vi "Set_Measurement_Conditions.vi"(3 "Simulate/Run":T3, 4 "Currently on Point":i32=11, 5 "Traverse line":T5 {"Row Duration (mins)" format="%#.1f"; "Row No" min=0; "Trace Gas Concentration (%)" min=0.0 format="%#.2f"; "Emission Rate (l/min)" format="%#.2f"; "Tunnel Speed" format="%#.2f"; "Start X" format="%#.2f"; "Start Y" format="%#.2f"; "Start Z" format="%#.2f"; "End X" format="%#.2f"; "End Y" format="%#.2f"; "End Z" format="%#.2f"; "Averaging time (min)" min=0.0 format="%#.2f"}) -> (0 "Status Cluster":T1)   [LabVIEW 2010]
uses:
  Traverse_cluster.ctl
  Spacing.ctl
  Controls/Multi_run_mode.ctl
  Execute_case.ctl
  Controls/User_Specific_mode.ctl
  Status_Cluster.ctl
  Multi_Run_Status.ctl
  ADAM Client/Sub VIs/ADAM Controls/Client_Source_Status.ctl
  Globals/Preference_global.vi
  Globals/Extra_Commands_Global.vi
panel:
  out "Heaters On?":bool
  out "Time Source Started":dbl
  out "Execute Case":T4=enum."Set All Conditions"
  # "X           Y            Z"
  # "Start"
  # "End"
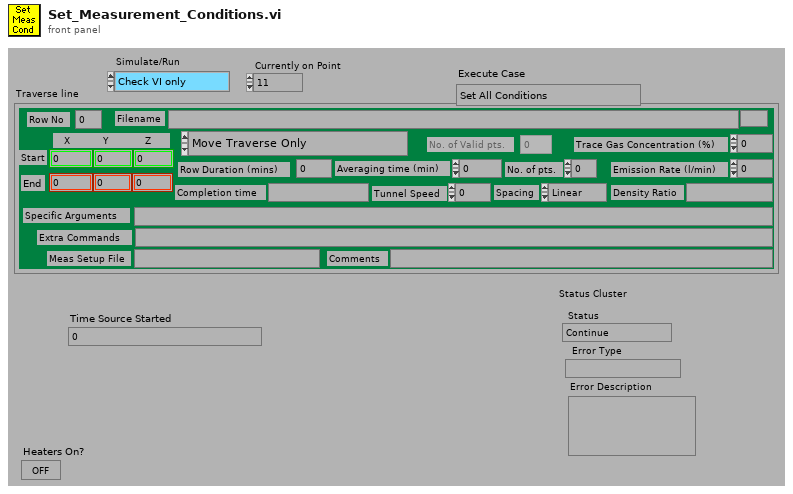
[diagram p1: front panel]
types:
  T1 = typedef "Status_Cluster.ctl" = cluster{"Status":T2, "Error Type":string, "Error Description":string}
  T2 = typedef "Multi_Run_Status.ctl" = enum16{"Continue", "Jump to Next Point", "Jump to Next Row", "Jump To Fall Back", "Terminate Run"}
  T3 = typedef "User_Specific_mode.ctl" = enum16{"Check VI only", "Run VI"}
  T4 = typedef "Execute_case.ctl" = enum16{"Start", "EnFlo Tunnel Check", "Set All Conditions", "Establish Exp Conditions", "The End"}
  T5 = typedef "Traverse_cluster.ctl" = cluster{"Start X":dbl, "Start Y":dbl, "Start Z":dbl, "End X":dbl, "End Y":dbl, "End Z":dbl, "No. of pts.":i32, "Spacing":T6, "Filename":path, "Tunnel Speed":dbl, "Averaging time (min)":dbl, "Extra Commands":string, "Specific Arguments":string, "Emission Rate (l/min)":dbl, "Trace Gas Concentration (%)":dbl, "Density Ratio":string, "Comments":string, "Row No":i32, "Row Type Selector":T7, "Completion time":string, "Row Duration (mins)":dbl, "No. of Valid pts.":i32, "Meas Setup File":string}
  T6 = typedef "Spacing.ctl" = enum16{"Linear", "Log", "Gauss", "Specified", "N/A"}
  T7 = typedef "Multi_run_mode.ctl" = enum16{"Move Traverse Only", "Set Tunnel Speed Only", "Set Source Only", "Set Measurement Conditions", "Single Measurement", "Vertical Profile", "Lateral Profile", "Longitudinal Profile", "Explore Volume", "Multi-Axis Profile", "Auto Calibrate", "Meas Fast FID Bkgnd", "Check Beam Power", "Scanning Valve Measurement", "Run VI Named:", "Set ADAM Ch", "Wait (minutes)", "Send Message", "Synchronize With:", "Fall Back to this Row", "Turn Off Row Repeating", "Blank Row"}
  T8 = typedef "Client_Source_Status.ctl" = enum16{"Not Using", "Using", "Must Have"}
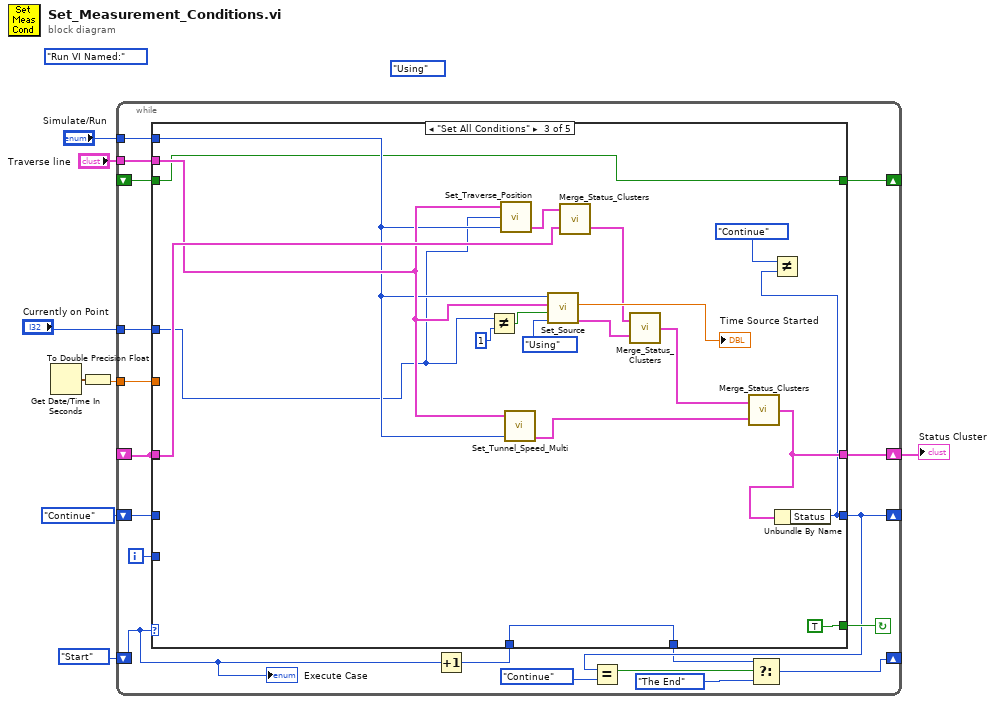
[diagram p0: block diagram]
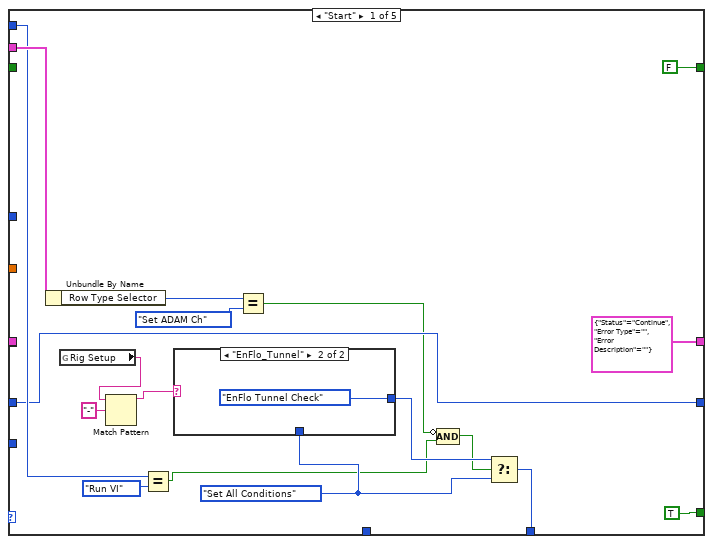
[diagram p2: hidden frame]
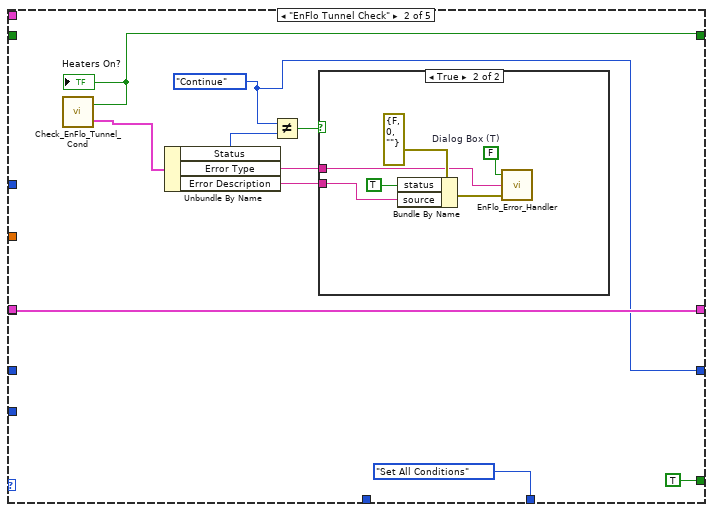
[diagram p4: hidden frame]
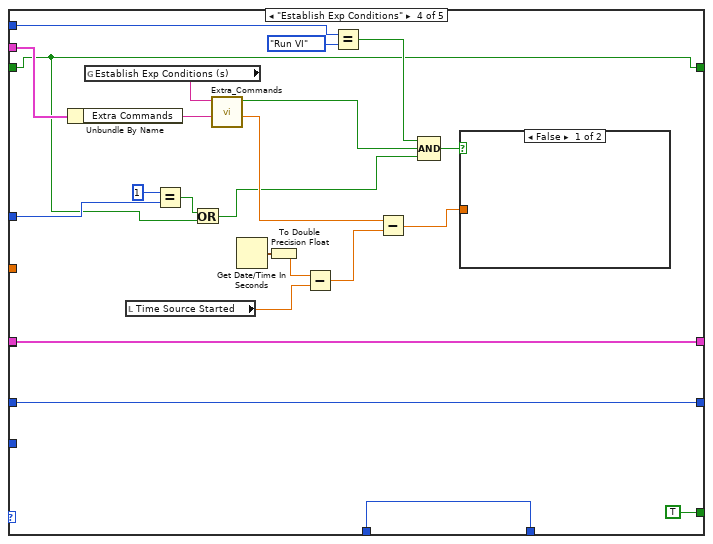
[diagram p6: hidden frame]
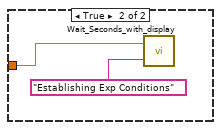
[diagram p7: hidden frame]
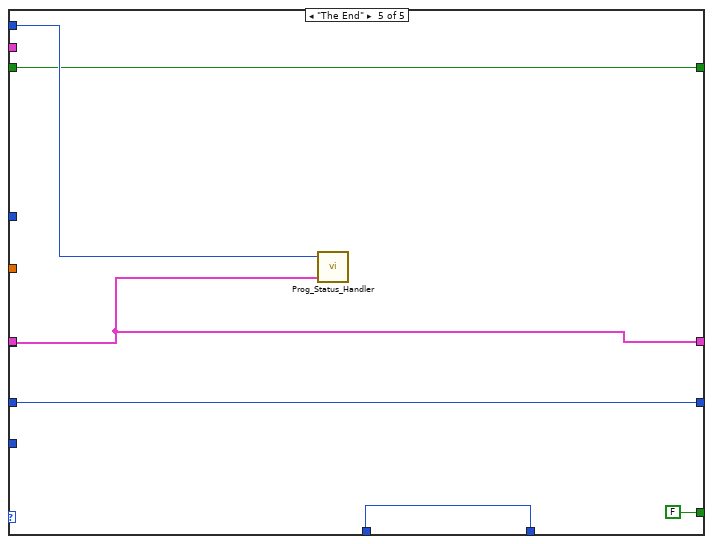
[diagram p8: hidden frame]
diagram:
  (unwired) Client_Source_Status."Using" ("Source Status")
  (unwired) Multi_run_mode."Run VI Named:" ("Mode")
  n1 = Get Date/Time In Seconds() -> (seconds since 1Jan1904=w1:timestamp)
  n2 = To Double Precision Float(number=w1) -> (double precision float=w2:dbl)
  n3 = while {
    tunnel: w2 -> [w12]
    tunnel: "Traverse line" -> [w13]
    tunnel: "Currently on Point" -> [w14]
    shift-left: _ -> [w15]
    shift-right: [w22] -> w4
    shift-left: Multi_Run_Status."Continue" ("Status") -> [w23]
    shift-right: [w21] -> _
    tunnel: "Simulate/Run" -> [w24]
    shift-left: Execute_case."Start" ("Execute Case") -> [w25]
    shift-right: [w17] -> _
    shift-right: [w10] -> _
    shift-left: _ -> [w9]
    i -> [w11]
    stop <- w27 continue-if-true
    n4 = Increment(x=w25) -> (x+1=w26:T4)
    n5 = case shown="\"Set All Conditions\"" w25 {
      tunnel: [TRUE TRUE TRUE TRUE FALSE] -> w27
      tunnel: w26 -> [_ _ w77 w96 w112]
      tunnel: w24 -> [w42 _ w73 w104 w110]
      tunnel: w23 -> [w38 _ _ w95 w111]
      tunnel: w15 -> [_ w52 w81 w94 w109]
      tunnel: [T1 {"Status"=enum."Continue", "Error Type"="", "Error Description"=""} ("Status Cluster") w52 w78 w94 w109] -> w22
      tunnel: [w38 w49 w74 w95 w111] -> w21
      tunnel: [w39 Execute_case."Set All Conditions" ("Execute Case") w77 w96 w112] -> w16
      tunnel: w15 -> [_ _ _ _ _]
      tunnel: w14 -> [_ _ w72 w92 _]
      tunnel: w13 -> [w44 _ w80 w103 _]
      tunnel: w12 -> [_ _ _ _ _]
      tunnel: w11 -> [_ _ _ _ _]
      tunnel: [FALSE w48 w69 w83 w108] -> w10
      tunnel: w9 -> [_ _ w69 w83 w108]
      frame "Start" {
        w40 = Execute_case."Set All Conditions" ("Execute Case")
        n6 = Unbundle By Name(w44) -> ("Row Type Selector"=w32:T7)
        n7 = global read "Preference_global.vi" "Rig Setup"() -> (w30:string)
        n8 = Match Pattern(string=w30, regular expression="-") -> (before substring=w29:string)  [unwired: 4 out]
        n9 = Equal?(x=w42, y=User_Specific_mode."Run VI" ("Simulate/Run")) -> (x = y?=w35:bool)
        n10 = case shown="\"EnFlo_Tunnel\"" w29 {
          tunnel: [w46 Execute_case."EnFlo Tunnel Check" ("Execute Case")] -> w41
          tunnel: w40 -> [w46 _]
          frame "Other", Default {
          }
          frame "EnFlo_Tunnel" {
          }
        }
        n11 = Equal?(x=w32, y=Multi_run_mode."Set ADAM Ch" ("Mode")) -> (x = y?=w36:bool)
        n12 = Compound Arithmetic op=AND(invert w36, w35) -> (w34:bool)
        n13 = Select(t=w41, s=w34, f=w40) -> (s? t:f=w39:T4)
      }
      frame "EnFlo Tunnel Check" {
        w49 = Multi_Run_Status."Continue" ("Status")
        n14 = call "Check_EnFlo_Tunnel_Cond.vi"() -> ("Status Cluster"=w55:T1, "Heaters On?"=w48:bool)  [unwired: 2 in]
        "Heaters On?" <- w48
        n15 = Unbundle By Name(w55) -> ("Status"=w51:T2, "Error Type"=w54:string, "Error Description"=w53:string)
        n16 = Not Equal?(x=w49, y=w51) -> (x != y?=w50:bool)
        n17 = case shown="True" w50 {
          tunnel: w54 -> [_ w59]
          tunnel: w53 -> [_ w58]
          frame False {
          }
          frame True {
            w61 = FALSE  # Dialog Box (T)
            n18 = Bundle By Name(cluster=errorcluster {"status"=FALSE, "code"=0, "source"=""} ("error in (no error)"), "status"=TRUE ("Bundle Element"), "source"=w58) -> (w62:errorcluster)
            n19 = call "EnFlo_Error_Handler.vi"("error in (no error)"=w62, "Error Type"=w59, "Dialog Box (T)"=w61) -> ()  [unwired: 3 out]
          }
        }
      }
      frame "Set All Conditions" {
        n20 = Not Equal?(x=w72, y=1) -> (x != y?=w66:bool)
        n21 = call "Set_Traverse_Position.vi"("Simulate/Run"=w73, "Currently on Point"=w72, "Traverse line"=w80) -> ("Status Cluster"=w64:T1)  [unwired: 2 out]
        n22 = call "Set_Tunnel_Speed_Multi.vi"("Simulate/Run"=w73, "Traverse line"=w80) -> ("Status Cluster"=w79:T1)  [unwired: 3 out]
        n23 = call "Set_Source.vi"("Source Status"=Client_Source_Status."Using", "Establish Exp Conditions"=w66, "Traverse line"=w80, "Simulate/Run"=w73) -> ("Status Cluster"=w65:T1, "Time Source Started"=→"Time Source Started":dbl)  [unwired: 4 out]
        n24 = call "Merge_Status_Clusters.vi"("Status Cluster 2"=w81, "Status Cluster 1"=w64) -> ("Status Cluster Out"=w71:T1)
        n25 = call "Merge_Status_Clusters.vi"("Status Cluster 2"=w65, "Status Cluster 1"=w71) -> ("Status Cluster Out"=w70:T1)
        n26 = call "Merge_Status_Clusters.vi"("Status Cluster 2"=w79, "Status Cluster 1"=w70) -> ("Status Cluster Out"=w78:T1)
        n27 = Unbundle By Name(w78) -> ("Status"=w74:T2)
        n28 = Not Equal?(x=Multi_Run_Status."Continue" ("Status"), y=w74) -> ()  [unwired: 1 out]
      }
      frame "Establish Exp Conditions" {
        n29 = Unbundle By Name(w103) -> ("Extra Commands"=w97:string)
        n30 = global read "Extra_Commands_Global.vi" "Establish Exp Conditions (s)"() -> (w102:string)
        n31 = local read "Time Source Started"() -> (w91:dbl)
        n32 = Equal?(x=1, y=w92) -> (x = y?=w85:bool)
        n33 = Or(x=w85, y=w83) -> (x .or. y?=w84:bool)
        n34 = call "Extra_Commands.vi"("String to Search"=w97, "Command"=w102) -> ("Numeric Value"=w89:dbl, "Command Found"=w99:bool)  [unwired: 1 in, 3 out]
        n35 = Get Date/Time In Seconds() -> (seconds since 1Jan1904=w86:timestamp)
        n36 = To Double Precision Float(number=w86) -> (double precision float=w90:dbl)
        n37 = Subtract(x=w90, y=w91) -> (x-y=w88:dbl)
        n38 = Equal?(x=w104, y=User_Specific_mode."Run VI" ("Simulate/Run")) -> (x = y?=w98:bool)
        n39 = Subtract(x=w89, y=w88) -> (x-y=w87:dbl)
        n40 = Compound Arithmetic op=AND(w98, w99, w84) -> (w100:bool)
        n41 = case shown="False" w100 {
          tunnel: w87 -> [_ w106]
          frame False {
          }
          frame True {
            n42 = call "Wait_Seconds_with_display.vi"("Message"="Establishing Exp Conditions", "Seconds to wait"=w106) -> ()  [unwired: 2 out]
          }
        }
      }
      frame "The End" {
        n43 = call "Prog_Status_Handler.vi"("Status Cluster"=w109, "Simulate/Run"=w110) -> ()  [unwired: 2 out]
      }
    }
    n44 = Equal?(x=w21, y=Multi_Run_Status."Continue" ("Status")) -> (x = y?=w19:bool)
    n45 = Select(t=w16, s=w19, f=Execute_case."The End" ("Execute Case")) -> (s? t:f=w17:T4)
    "Execute Case" <- w25
  }
  "Status Cluster" <- w4
